vi "COMI AD Get Digit.vi"(10 "ch":i32, 11 "hDevice":u32) -> (2 "function return":i16, 3 "hDevice out":u32)   [LabVIEW 2017, in "Comidll.lvlib"]
doc: "short (COMI_AD_GetDigit) (HANDLE hDevice, int ch);"
uses:
  <userlib>/Comidll/Comidll.lvlib
  <userlib>/Comidll/Comidll.dll
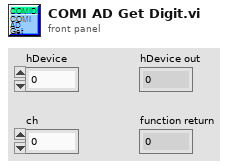
[diagram p1: front panel]
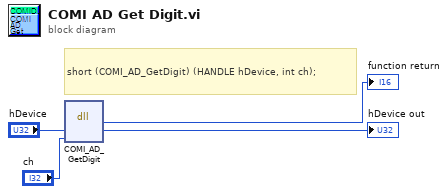
[diagram p0: block diagram]
diagram:
  # "short\t(COMI_AD_GetDigit) (HANDLE hDevice, int ch);"
  n1 = dll-call lib="C:/Program Files/National Instruments/LabVIEW 2017/user.lib/Comidll/Comidll.*" fn="COMI_AD_GetDigit"("hDevice"="hDevice", "ch"="ch") -> (→"function return":i16, "hDevice"=→"hDevice out":u32)  [unwired: 4 in, 2 out]
